vi "NR Configure ModAcc.vi"(0 "RFmx Handle In":refnum<k21>, 1 "Selector String":string, 5 "NR ModAcc Configuration":T1={"Measurement Length Unit"=1, "Measurement Offset"=0.0, "Measurement Length"=1.0, "EVM Unit"=0, "Averaging Enabled"=0, "Averaging Count"=10, "ModAcc Sync Mode"=1} {"ModAcc Sync Mode" items=["Slot"=1, "Frame"=5]; "Averaging Enabled" items=["False", "True"]; "EVM Unit" items=["Percentage", "dB"]; "Measurement Length Unit" items=["Slot"=1, "Subframe"=3, "Time"=6]}, 11 "error in (no error)":errorcluster) -> (4 "RFmx Handle Out":refnum<k21>, 15 "error out":errorcluster)   [LabVIEW 2019, in "RFmxNR.lvlib"]
doc: "Configures common settings for the ModAcc measurement and selects the measurement."
uses:
  RFmxNR.lvlib
  Typedefs/NR ModAcc Configuration.ctl
  <vilib>/RFmx/NR/mx/RFmxNR.llb/RFmxNR Select Measurement (Single).vi
  <resource>/objmgr/RFmxNR.rc
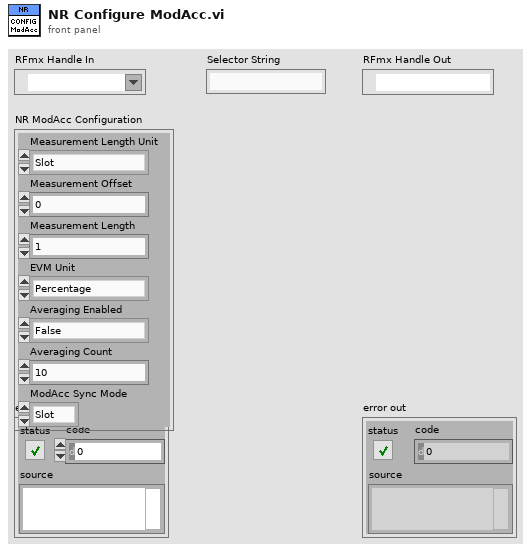
[diagram p1: front panel]
types:
  T1 = typedef "RFmxNR.lvlib/NR ModAcc Configuration.ctl" = cluster{"Measurement Length Unit":i32, "Measurement Offset":dbl, "Measurement Length":dbl, "EVM Unit":i32, "Averaging Enabled":i32, "Averaging Count":i32, "ModAcc Sync Mode":i32}
  T2 = enum16{"ModAcc", "SEM", "ACP", "CHP", "OBW", "PVT"}
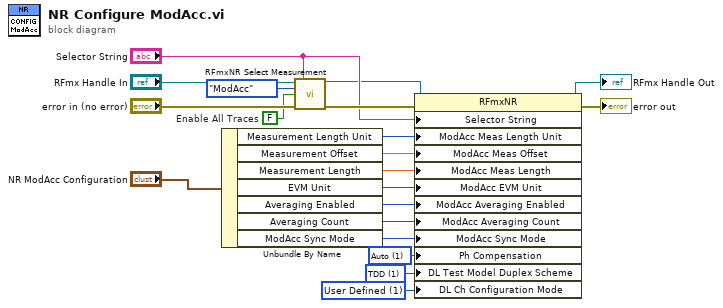
[diagram p0: block diagram]
diagram:
  w1 = 1 items=["User Defined"=1, "Test Model"=2] ("DL Ch Configuration Mode")
  w2 = 1 items=["FDD", "TDD"] ("DL Test Model Duplex Scheme")
  w3 = 1 items=["Disabled", "Auto", "User Defined"] ("Ph Compensation")
  w5 = FALSE  # Enable All Traces
  n1 = Unbundle By Name("NR ModAcc Configuration") -> ("Measurement Length Unit"=w16:i32, "Measurement Offset"=w15:dbl, "Measurement Length"=w14:dbl, "EVM Unit"=w13:i32, "Averaging Enabled"=w12:i32, "Averaging Count"=w11:i32, "ModAcc Sync Mode"=w4:i32)
  n2 = call-poly <vilib>:"RFmxNR Select Measurement.vi"("Instrument Handle In"="RFmx Handle In", "Selector String"="Selector String", "Measurement"=T2."ModAcc", "Enable All Traces"=w5, "error in (no error)"="error in (no error)") -> ("Instrument Handle Out"=w8:refnum<k21>, "error out"=w18:errorcluster)  [unwired: 9 in]
  n3 = property class="RFmxNR"(reference=w8, error in=w18, "Selector String"="Selector String", "ModAcc Meas Length Unit"=w16, "ModAcc Meas Offset"=w15, "ModAcc Meas Length"=w14, "ModAcc EVM Unit"=w13, "ModAcc Averaging Enabled"=w12, "ModAcc Averaging Count"=w11, "ModAcc Sync Mode"=w4, "Ph Compensation"=w3, "DL Test Model Duplex Scheme"=w2, "DL Ch Configuration Mode"=w1) -> (reference out=→"RFmx Handle Out":refnum<k21>, error out=→"error out":errorcluster)
